vi "nanocal -- defaut parameter manager -- V1.vi"(7 "action":T2=enum."update", 8 "T":dbl=0.269210160049 format="%#_13g", 9 "internal map":map{T1, dbl[]}(c390), 10 "what":T1) -> (1 "number":dbl)   [LabVIEW 2020]
uses:
  3-lorentzian-parameters.ctl
  nanocal -- defaut parameter manager action-- V1.ctl
  <vilib>/Analysis/NI_AALPro.lvlib
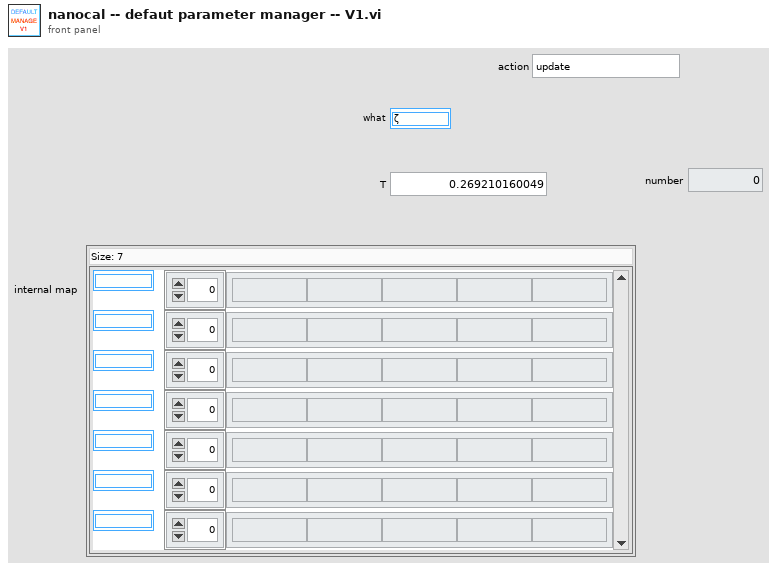
[diagram p1: front panel]
types:
  T1 = typedef "3-lorentzian-parameters.ctl" = enum16{"ζ", "τ1", "τS", "τN", "τC", "κ0", "m1", "m2", "m3", "T (K)", "B (T)", "θ (deg)", "side (S|R)", "set of (B|T)"}
  T2 = typedef "nanocal -- defaut parameter manager action-- V1.ctl" = enum16{"get logarithmic interp", "update", "get linear interp"}
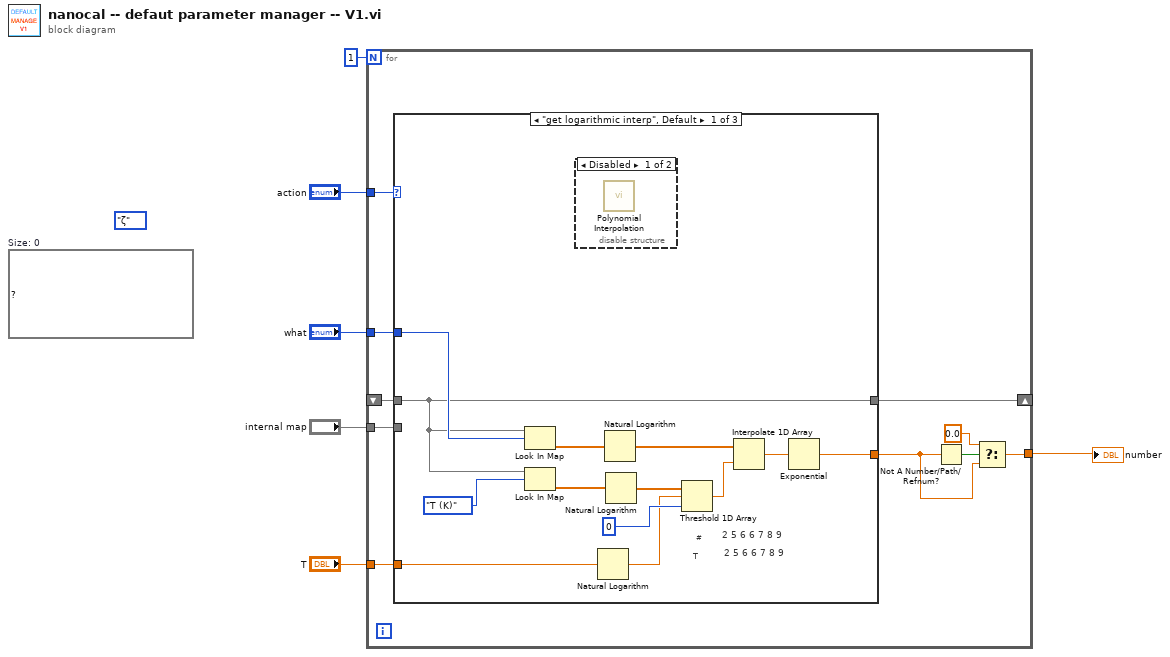
[diagram p0: block diagram]
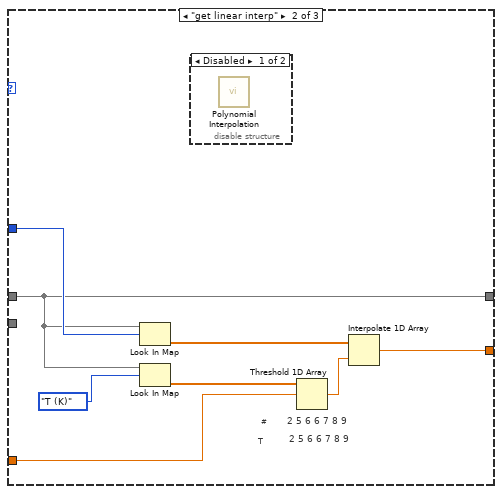
[diagram p3: hidden frame]
diagram:
  (unwired) map{T1, dbl[]} {}  # Size: 0
  (unwired) 3-lorentzian-parameters."ζ" ("Plost: sweep window")
  n1 = for {
    N: 1 -> [_]
    tunnel: "action" -> [w16]
    shift-right: [w15] -> _
    shift-left: _ -> [w14]
    tunnel: "internal map" -> [w13]
    tunnel: "what" -> [w12]
    tunnel: "T" -> [w11]
    tunnel: [w9] -> w2
    n2 = case shown="\"get logarithmic interp\", Default" w16 {
      tunnel: [w27 w35 w38] -> w15
      tunnel: w14 -> [w27 w35 _]
      tunnel: w13 -> [_ _ w38]
      tunnel: w12 -> [w29 w37 _]
      tunnel: w11 -> [w18 w34 _]
      tunnel: [w20 w31 _] -> w7
      frame "get logarithmic interp", Default {
        # "#"
        # "T"
        # "2 5 6 6 7 8 9"
        # "2 5 6 6 7 8 9"
        n3 = Look In Map(map=w27, key=w29) -> (value=w26:dbl[])  [unwired: 1 in, 1 out]
        n4 = Look In Map(map=w27, key=3-lorentzian-parameters."T (K)" ("Plost: sweep window")) -> (value=w25:dbl[])  [unwired: 1 in, 1 out]
        n5 = disable-structure shown="Disabled" {
          frame Disabled {
            n6 = call <vilib>:"Polynomial Interpolation.vi"() -> ()  [unwired: 3 in, 3 out]
          }
          frame Enabled {
          }
        }
        n7 = Natural Logarithm(1:w18) -> (0:w17:dbl)
        n8 = Natural Logarithm(1:w26) -> (0:w22:dbl[])
        n9 = Natural Logarithm(1:w25) -> (0:w24:dbl[])
        n10 = Threshold 1D Array(1:0 ("start index (0)"), 2:w17, 3:w24) -> (0:w23:dbl)
        n11 = Interpolate 1D Array(1:w23, 2:w22) -> (0:w21:dbl)
        n12 = Exponential(1:w21) -> (0:w20:dbl)
      }
      frame "get linear interp" {
        # "#"
        # "T"
        # "2 5 6 6 7 8 9"
        # "2 5 6 6 7 8 9"
        n13 = Look In Map(map=w35, key=w37) -> (value=w32:dbl[])  [unwired: 1 in, 1 out]
        n14 = Look In Map(map=w35, key=3-lorentzian-parameters."T (K)" ("Plost: sweep window")) -> (value=w30:dbl[])  [unwired: 1 in, 1 out]
        n15 = disable-structure shown="Disabled" {
          frame Disabled {
            n16 = call <vilib>:"Polynomial Interpolation.vi"() -> ()  [unwired: 3 in, 3 out]
          }
          frame Enabled {
          }
        }
        n17 = Threshold 1D Array(2:w34, 3:w30) -> (0:w33:dbl)  [unwired: 1 in]
        n18 = Interpolate 1D Array(1:w33, 2:w32) -> (0:w31:dbl)
      }
      frame "update" {
      }
    }
    n19 = Not A Number/Path/Refnum?(number/path/refnum=w7) -> (NaN/Path/Refnum?=w10:bool)
    n20 = Select(t=0.0, s=w10, f=w7) -> (s? t:f=w9:dbl)
  }
  "number" <- w2
